vi "Write Command Core.vi"(8 "error in (no error)":errorcluster, 10 "Message":refnum<class "Message Interface.lvclass">, 11 "Websocket Client Handler in":refnum<class "Websocket Client Handler.lvclass">) -> (0 "error out":errorcluster, 2 "JSON String":string, 3 "Websocket Client Handler out":refnum<class "Websocket Client Handler.lvclass">)   [LabVIEW 2016, in "Stream Mediator.lvlib" / "Websocket Client Handler.lvclass"]
doc: "--\nCopyright © 2017 Composed SystemsI All rights reserved.\n\nAuthor: Jon McBee <jon.mcbee@composed.io>\n\nThis library is provided \"AS IS\" ,WITHOUT WARRANTIES OR\nCONDITIONS OF ANY KIND, either express or implied.\n\nComposed Systems -- composed.io\n\nStream 0.0.1.1\nJon McBee - Composed Systems\nCopyright (c) 2017, Composed Systems"
uses:
  <userlib>/Composed Systems/Stream/Mediator/Classes/Websocket Client Handler Actor/Websocket Client Handler/Websocket Client Handler.lvclass
  <userlib>/Composed Systems/Stream/Mediator/Classes/Message Interface/Message Interface.lvclass
  <vilib>/addons/_JKI.lib/Serialization/JSON/JKI JSON Serialization.lvlib
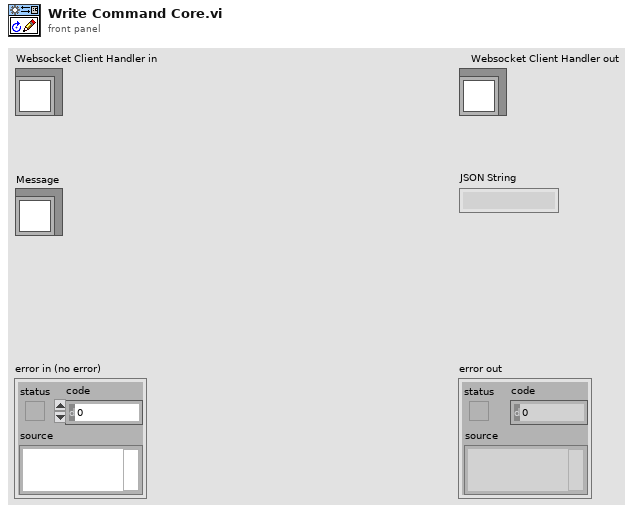
[diagram p1: front panel]
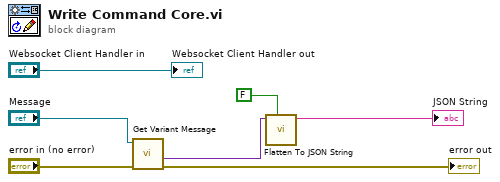
[diagram p0: block diagram]
diagram:
  n1 = call-dynamic "Get Variant Message.vi"("error in (no error)"="error in (no error)", "Message Interface in"="Message") -> ("error out"=→"error out":errorcluster, "Value"=w3:variant)  [unwired: 6 in, 2 out]
  n2 = call <vilib>:"Flatten To JSON String.vi"("Multiline (T)"=FALSE, "Variant"=w3) -> ("JSON String"=→"JSON String":string)  [unwired: 8 in, 1 out]
  "Websocket Client Handler out" <- "Websocket Client Handler in"
